vi "PreprocessMonitors.vi"(11 "MessageQueues":T1) -> (1 "Array 3":waveform(dbl)[](array[waveform]), 4 "Waveform":waveform(dbl))   [LabVIEW 2020]
uses:
  MessageQueues.ctl
  <vilib>/httpClient/ClientHandle.ctl
  <vilib>/httpClient/LabVIEWHTTPClient.lvlib
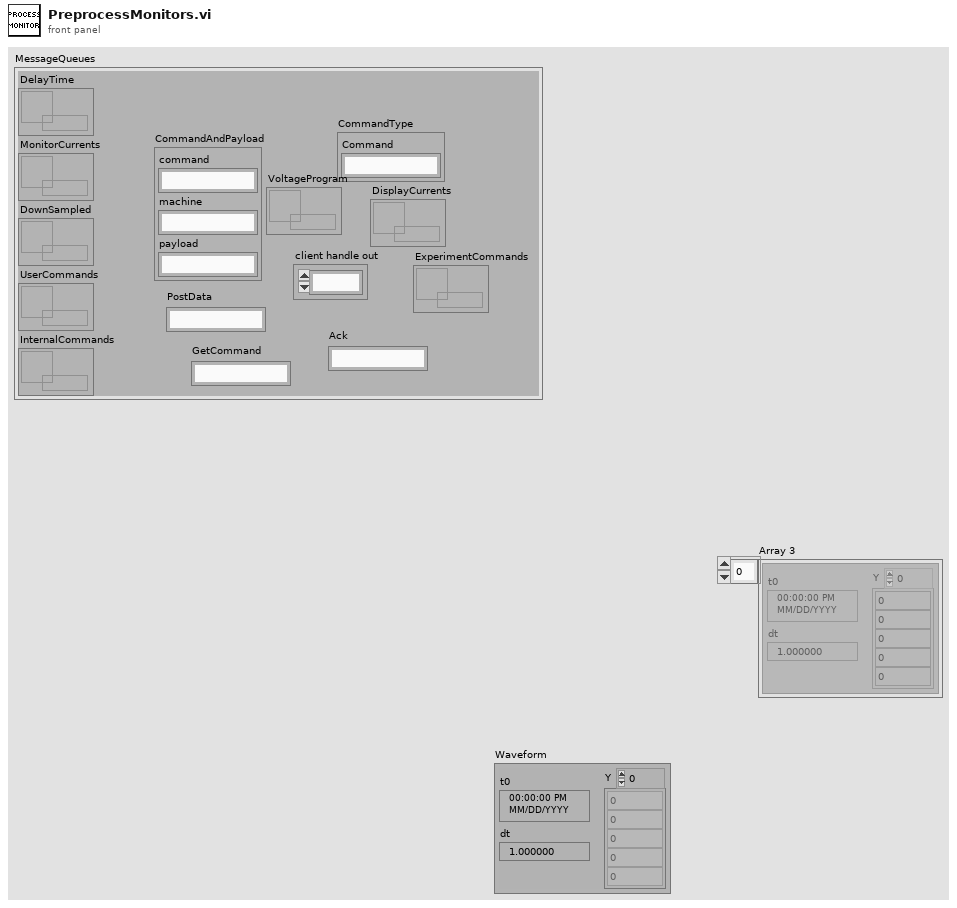
[diagram p1: front panel]
types:
  T1 = typedef "MessageQueues.ctl" = cluster{"DelayTime":refnum<queue>, "MonitorCurrents":refnum<queue>, "DownSampled":refnum<queue>, "UserCommands":refnum<queue>, "InternalCommands":refnum<queue>, "CommandType":cluster{"Command":string}, "CommandAndPayload":cluster{"command":string, "machine":string, "payload":string}, "client handle out":T2, "PostData":string, "GetCommand":string, "Ack":string, "VoltageProgram":refnum<queue>, "ExperimentCommands":refnum<queue>, "DisplayCurrents":refnum<queue>}
  T2 = typedef "LabVIEWHTTPClient.lvlib/ClientHandle.ctl" = refnum<k1>
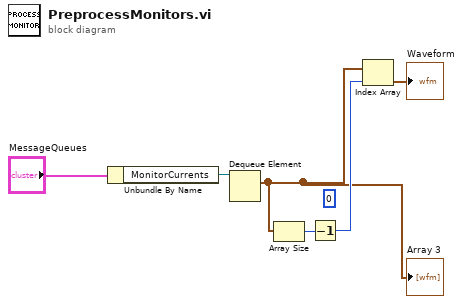
[diagram p0: block diagram]
diagram:
  (unwired) 0 ("index")
  n1 = Unbundle By Name("MessageQueues") -> ("MonitorCurrents"=w5:refnum<queue>)
  n2 = Dequeue Element(queue=w5) -> (element=w1:waveform(dbl)[])  [unwired: 2 in, 3 out]
  "Array 3" <- w1
  n3 = Array Size(array=w1) -> (size(s)=w2:i32)
  n4 = Decrement(x=w2) -> (x-1=w3:i32)
  n5 = Index Array(array=w1, index=w3) -> (element=→"Waveform":waveform(dbl))
